vi "Channel_Name_Options.vi"(0 "All Channel Names":string[](array[string]), 1 "Data string":string, 2 "Ignore When":string[][](array[string]), 3 "Reading Filename":path, 5 "Template Names":string[](array[string]), 9 "Start of data (bytes)":i32, 11 "Maths In":string[](array[string]), 12 "Name Options In":string[][](array[string]), 13 "Filetype":string) -> (4 "Channels to find":string[](array[string]), 6 "Valid Channel Options":string[][](array[string]), 15 "Name Options Out":string[][](array[string]))   [LabVIEW 2013]
uses:
  Results_plotter_Global.vi
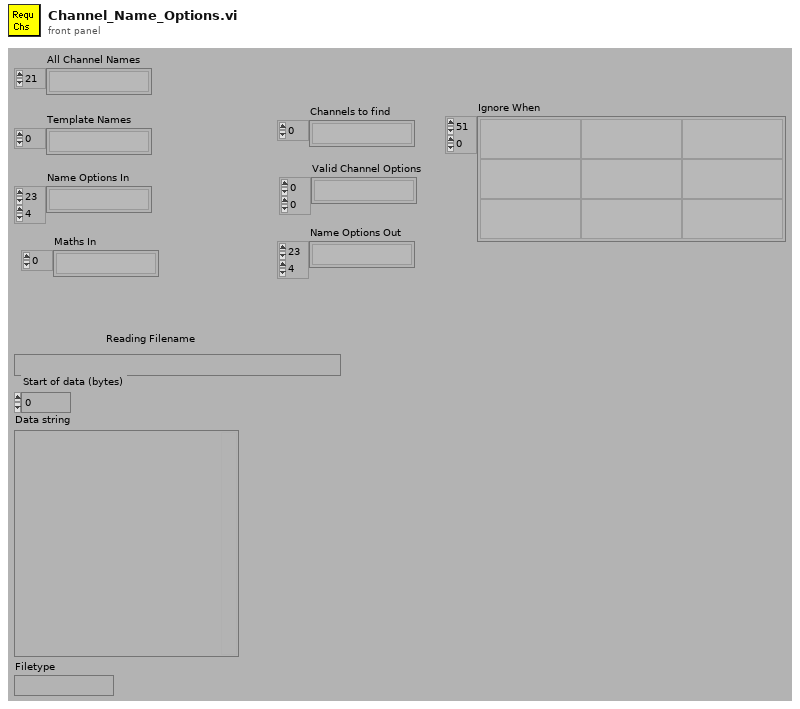
[diagram p1: front panel]
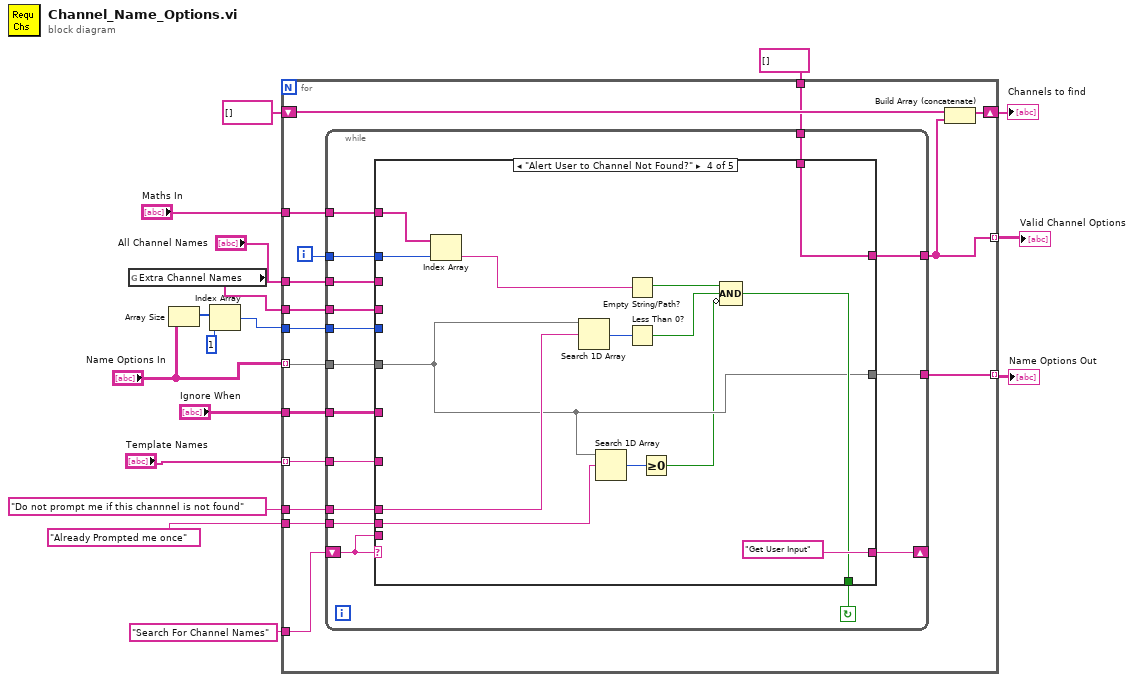
[diagram p0: block diagram]
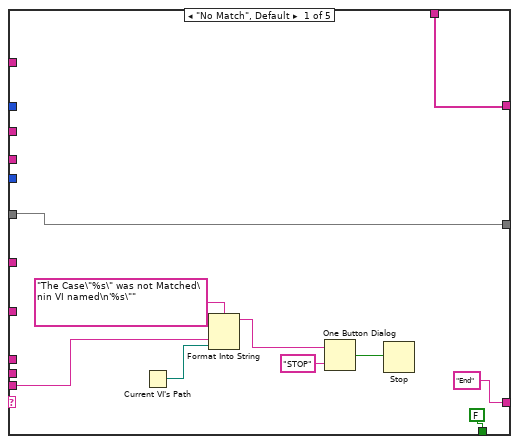
[diagram p2: hidden frame]
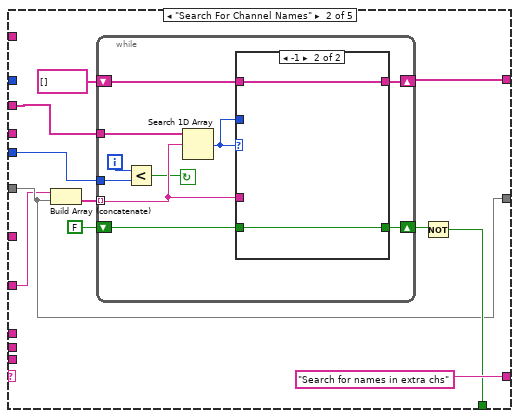
[diagram p3: hidden frame]
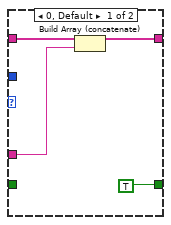
[diagram p4: hidden frame]
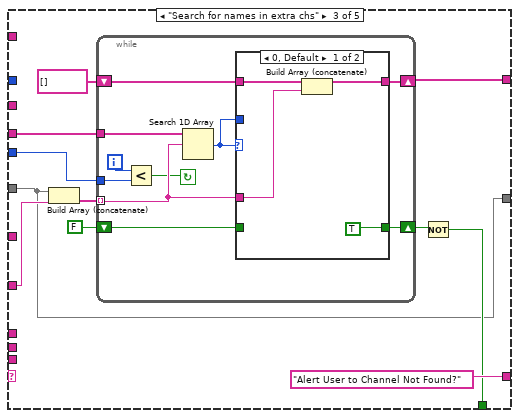
[diagram p5: hidden frame]
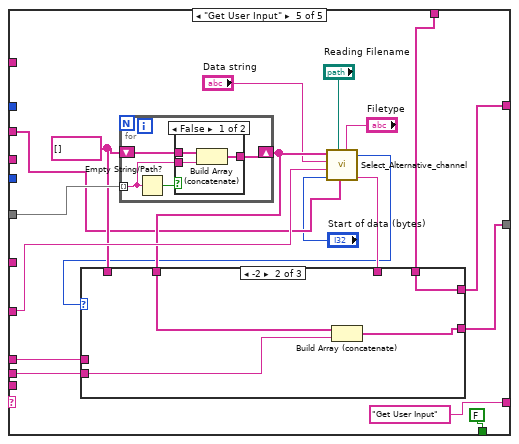
[diagram p7: hidden frame]
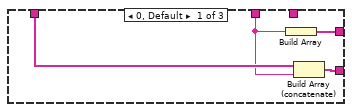
[diagram p8: hidden frame]
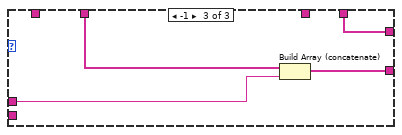
[diagram p9: hidden frame]
diagram:
  n1 = global read "Results_plotter_Global.vi" "Extra Channel Names"() -> (w4:string[])
  n2 = Array Size(array="Name Options In") -> (size(s)=w15:i32[])
  n3 = Index Array(array=w15, index=1 ("Index")) -> (element=w12:i32)
  n4 = for {
    tunnel: "All Channel Names" -> [w33]
    tunnel: "Name Options In" -> [w31] mode=indexing
    tunnel: w12 -> [w32]
    tunnel: [w22] -> w9 mode=indexing
    tunnel: "Template Names" -> [w30] mode=indexing
    tunnel: [w29] -> w17 mode=indexing
    tunnel: "Do not prompt me if this channnel is not found" -> [w28]
    tunnel: "Maths In" -> [w27]
    tunnel: "Search For Channel Names" -> [w25]
    shift-right: [w23] -> w7
    shift-left: string[] [] -> [w24]
    tunnel: string[] [] -> [w21]
    tunnel: w4 -> [w20]
    tunnel: "Already Prompted me once" -> [w19]
    tunnel: "Ignore When" -> [w18]
    i -> [w26]
    n5 = while {
      tunnel: w20 -> [w36]
      tunnel: w21 -> [w37]
      tunnel: [w38] -> w22
      tunnel: w26 -> [w39]
      tunnel: w27 -> [w41]
      tunnel: w28 -> [w42]
      tunnel: [w43] -> w29
      tunnel: w30 -> [w44]
      tunnel: w31 -> [w47]
      tunnel: w32 -> [w48]
      tunnel: w33 -> [w49]
      shift-left: w25 -> [w40]
      shift-right: [w45] -> _
      tunnel: w19 -> [w35]
      tunnel: w18 -> [w34]
      stop <- w46 continue-if-true
      n6 = case shown="\"Alert User to Channel Not Found?\"" w40 {
        tunnel: w49 -> [_ w61 _ _ w133]
        tunnel: w48 -> [_ w70 w97 _ _]
        tunnel: w47 -> [w51 w62 w88 w117 w145]
        tunnel: [w50 w66 w93 w118 w142] -> w38
        tunnel: [FALSE w64 w91 w122 FALSE] -> w46
        tunnel: ["End" "Search for names in extra chs" "Alert User to Channel Not Found?" "Get User Input" "Get User Input"] -> w45
        tunnel: w44 -> [_ w60 w90 _ w141]
        tunnel: [w51 w62 w88 w117 w143] -> w43
        tunnel: w42 -> [_ _ _ w126 w129]
        tunnel: w41 -> [_ _ _ w121 _]
        tunnel: w40 -> [w54 _ _ _ _]
        tunnel: w39 -> [_ _ _ w120 _]
        tunnel: w37 -> [w50 _ _ w118 w136]
        tunnel: w36 -> [_ _ w87 _ _]
        tunnel: w35 -> [_ _ _ w116 w128]
        tunnel: w34 -> [_ _ _ _ _]
        frame "No Match", Default {
          n7 = Current VI's Path() -> (path=w55:path)
          n8 = Format Into String(format string="The Case\"%s\" was not Matched\nin VI named\n'%s\"" ("Format String"), w54, w55) -> (resulting string=w58:string)  [unwired: 2 in, 1 out]
          n9 = One Button Dialog(message=w58, button name ("OK")="STOP") -> (true=w56:bool)
          n10 = Stop(stop? (T)=w56) -> ()
        }
        frame "Search For Channel Names" {
          n11 = Build Array (concatenate)(w60, w62) -> (w63:string[])
          n12 = while {
            shift-left: string[] [] -> [w72]
            shift-right: [w75] -> w66
            shift-left: FALSE ("index of element") -> [w73]
            shift-right: [w74] -> w65
            tunnel: w63 -> [w77] mode=indexing
            tunnel: w70 -> [w78]
            tunnel: w61 -> [w80]
            i -> [w79]
            stop <- w71 continue-if-true
            n13 = Less?(x=w79, y=w78) -> (x < y?=w71:bool)
            n14 = Search 1D Array(1D array=w80, element=w77) -> (index of element=w76:i32)  [unwired: 1 out]
            n15 = case shown="-1" w76 {
              tunnel: w77 -> [w82 _]
              tunnel: w76 -> [_ _]
              tunnel: [w83 w85] -> w75
              tunnel: [TRUE w86] -> w74
              tunnel: w73 -> [_ w86]
              tunnel: w72 -> [w84 w85]
              frame 0, Default {
                n16 = Build Array (concatenate)(w84, w82) -> (w83:string[])
              }
              frame -1 {
              }
            }
          }
          n17 = Not(x=w65) -> (.not. x?=w64:bool)
        }
        frame "Search for names in extra chs" {
          n18 = Build Array (concatenate)(w88, w90) -> (w89:string[])
          n19 = while {
            shift-left: string[] [] -> [w99]
            shift-right: [w102] -> w93
            shift-left: FALSE ("index of element") -> [w100]
            shift-right: [w101] -> w92
            tunnel: w89 -> [w104] mode=indexing
            tunnel: w97 -> [w105]
            tunnel: w87 -> [w107]
            i -> [w106]
            stop <- w98 continue-if-true
            n20 = Less?(x=w106, y=w105) -> (x < y?=w98:bool)
            n21 = Search 1D Array(1D array=w107, element=w104) -> (index of element=w103:i32)  [unwired: 1 out]
            n22 = case shown="0, Default" w103 {
              tunnel: w104 -> [w109 _]
              tunnel: w103 -> [_ _]
              tunnel: [w110 w112] -> w102
              tunnel: [TRUE w113] -> w101
              tunnel: w100 -> [_ w113]
              tunnel: w99 -> [w111 w112]
              frame 0, Default {
                n23 = Build Array (concatenate)(w111, w109) -> (w110:string[])
              }
              frame -1 {
              }
            }
          }
          n24 = Not(x=w92) -> (.not. x?=w91:bool)
        }
        frame "Alert User to Channel Not Found?" {
          n25 = Index Array(array=w121, index=w120) -> (element=w119:string)
          n26 = Search 1D Array(1D array=w117, element=w126) -> (index of element=w127:i32)  [unwired: 1 out]
          n27 = Search 1D Array(1D array=w117, element=w116) -> (index of element=w115:i32)  [unwired: 1 out]
          n28 = Empty String/Path?(string/path=w119) -> (empty?=w124:bool)
          n29 = Less Than 0?(x=w127) -> (x < 0?=w123:bool)
          n30 = Greater Or Equal To 0?(x=w115) -> (x >= 0?=w114:bool)
          n31 = Compound Arithmetic op=AND(w124, w123, invert w114) -> (w122:bool)
        }
        frame "Get User Input" {
          w138 = string[] []
          n32 = for {
            shift-right: [w158] -> w140
            shift-left: w138 -> [w160]
            tunnel: w145 -> [w159] mode=indexing
            n33 = Empty String/Path?(string/path=w159) -> (empty?=w161:bool)
            n34 = case shown="False" w161 {
              tunnel: w160 -> [w164 w165]
              tunnel: [w163 w165] -> w158
              tunnel: w159 -> [w162 _]
              frame False {
                n35 = Build Array (concatenate)(w164, w162) -> (w163:string[])
              }
              frame True {
              }
            }
          }
          n36 = call "Select_Alternative_channel.vi"("Filetype"="Filetype", "All Tabulated Channels"=w133, "Reading Filename"="Reading Filename", "Start of data (bytes)"="Start of data (bytes)", "Template Channel Name"=w141, "Data string"="Data string", "Previous Channels used"=w140) -> ("Choosen Channel"=w139:string, "Selected Index"=w135:i32)  [unwired: 2 out]
          n37 = case shown="-2" w135 {
            tunnel: [w149 w151 w157] -> w143
            tunnel: [w146 w153 w156] -> w142
            tunnel: w140 -> [w148 w152 w155]
            tunnel: w139 -> [w147 _ _]
            tunnel: w138 -> [_ _ _]
            tunnel: w136 -> [_ w153 w156]
            tunnel: w129 -> [_ _ w154]
            tunnel: w128 -> [_ w150 _]
            frame 0, Default {
              n38 = Build Array(w147) -> (w146:string[])
              n39 = Build Array (concatenate)(w148, w147) -> (w149:string[])
            }
            frame -2 {
              n40 = Build Array (concatenate)(w152, w150) -> (w151:string[])
            }
            frame -1 {
              n41 = Build Array (concatenate)(w155, w154) -> (w157:string[])
            }
          }
        }
      }
    }
    n42 = Build Array (concatenate)(w24, w22) -> (w23:string[])
  }
  "Name Options Out" <- w17
  "Valid Channel Options" <- w9
  "Channels to find" <- w7
